vi "Untitled 3.vi"(4 "String":refnum<vi>, 5 "Event Data":T1, 6 "Control Ref":refnum<k24>, 7 "Event Common Data":T2) -> ()   [LabVIEW 2014]
uses:
  U:/Visual Studio 2015/Projects/Exemple/Exemple/bin/Debug/Exemple.dll
  bin/Debug/Exemple.dll
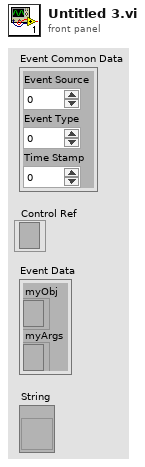
[diagram p1: front panel]
types:
  T1 = cluster{"myObj":refnum<k24>, "myArgs":refnum<k24>}
  T2 = cluster{"Event Source":i32, "Event Type":u32, "Time Stamp":u32}
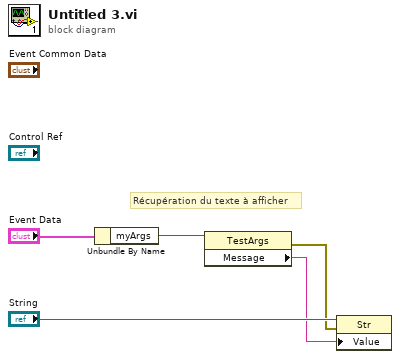
[diagram p0: block diagram]
diagram:
  # "Récupération du texte à afficher"
  n1 = Unbundle By Name("Event Data") -> ("myArgs"=w4:refnum<k24>)
  n2 = property class="TestArgs"(reference=w4) -> (error out=w1:errorcluster, "Message"=w2:string)  [unwired: 1 in, 1 out]
  n3 = property class="Str"(reference="String", error in=w1, "Value"=w2) -> ()  [unwired: 2 out]
